vi "Get Resources.vi"(8 "error in (no error)":errorcluster, 11 "id":i32) -> (0 "error out":errorcluster, 3 "resources":T1[](array[typedef]))   [LabVIEW 2020, in "MCP Server.lvlib"]
uses:
  MCP Server.lvlib
  resource data.ctl
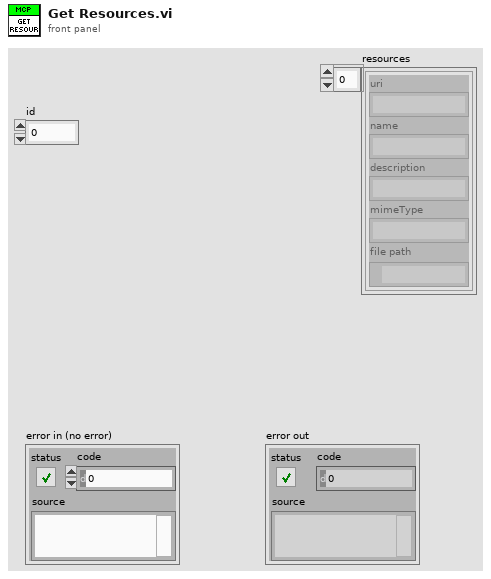
[diagram p1: front panel]
types:
  T1 = typedef "MCP Server.lvlib/resource data.ctl" = cluster{"uri":string, "name":string, "description":string, "mimeType":string, "file path":path}
  T2 = typedef "MCP Server.lvlib/Server Data.ctl" = cluster{"Name":string, "Description":string, "Tools":T3[], "Parameters":string[][], "Logging Info":T6, "User Events":T7, "Prompts":T8[], "resources":T1[], "HTTP Server":refnum<class "Server.lvclass">}
  T3 = typedef "MCP Server.lvlib/Tool Data.ctl" = cluster{"Name":string, "Description":string, "Ignored":string[], "inputs":T4[], "outputs":T5[], "VI Refnum":refnum<vi>}
  T4 = typedef "MCP Server.lvlib/Input Parameter.ctl" = cluster{"name":string, "type":string, "description":string, "required":bool, "raw name":string}
  T5 = typedef "MCP Server.lvlib/Output Parameter.ctl" = cluster{"name":string, "description":string, "type":string, "raw name":string}
  T6 = typedef "MCP Server.lvlib/Logging.ctl" = cluster{"Log":string[], "Max Length":i32}
  T7 = typedef "MCP Server.lvlib/User Events.ctl" = cluster{"onError":refnum<user-event>, "onRpc":refnum<user-event>}
  T8 = typedef "MCP Server.lvlib/Prompt Data.ctl" = cluster{"name":string, "description":string, "arguments":T9[], "return terminal name":string, "results description":string, "VI Refnum":refnum<vi>}
  T9 = typedef "MCP Server.lvlib/Prompt Argument.ctl" = cluster{"name":string, "description":string, "required":bool, "raw_name":string}
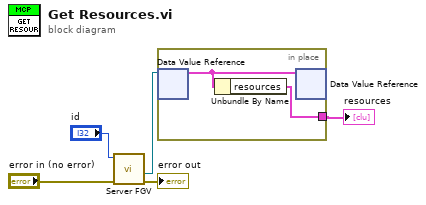
[diagram p0: block diagram]
diagram:
  n1 = call "Server FGV.vi"("error in"="error in (no error)", "id"="id") -> ("error out"=→"error out":errorcluster, "server reference"=w5:refnum<data-value>)  [unwired: 5 in, 3 out]
  n2 = in-place {
    in-place-border: [w7] -> w1
    n3 = in-place-dvr #1(w5) -> (w6:T2)  [unwired: 1 out]
    n4 = Unbundle By Name(w6) -> ("resources"=w7:T1[])
    n5 = in-place-dvr #1(w6) -> ()  [unwired: 2 out]
  }
  "resources" <- w1
